vi "Get Blob Properties.vi"(8 "error in (no error)":errorcluster, 9 "Blob":string, 10 "Container":string, 11 "Azure Session in":refnum<class "Session.lvclass">) -> (0 "error out":errorcluster, 2 "Blob Properties":T1[](array[typedef]), 3 "Azure Session out":refnum<class "Session.lvclass">)   [LabVIEW 2015, in "NI_Azure_Blob.lvlib"]
doc: "Returns all system properties and user-defined metadata on the blob."
uses:
  NI_Azure_Blob.lvlib
  Core/Session/Session.lvclass
  Core/Name Value Pair.ctl
  Core/Session/Session.lvclass/Session.ctl
  Core/Session/Write HTTP Verb.vi
  Core/Session/Write URL Suffix.vi
  Core/NI_Azure_Core.lvlib
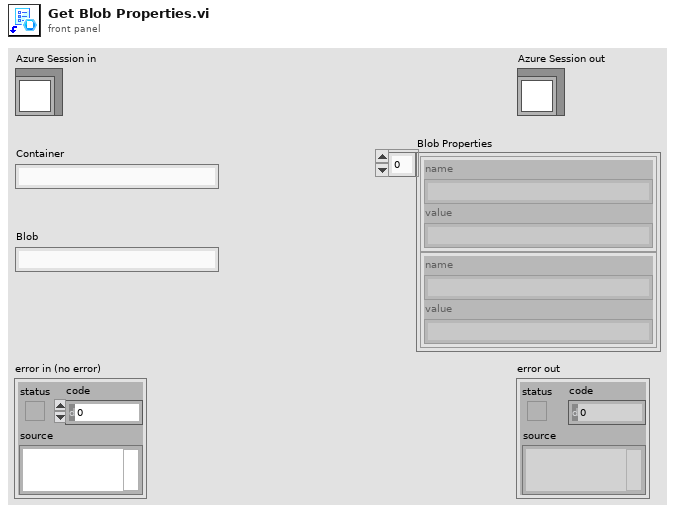
[diagram p1: front panel]
types:
  T1 = typedef "NI_Azure_Core.lvlib/Name Value Pair.ctl" = cluster{"name":string, "value":string}
  T2 = typedef "NI_Azure_Core.lvlib/Response.ctl" = cluster{"Headers":string, "Body":string}
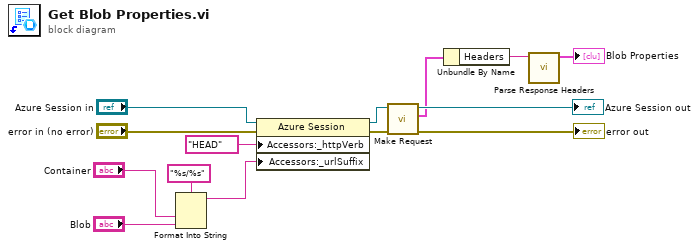
[diagram p0: block diagram]
diagram:
  n1 = Format Into String(format string="%s/%s", "Container", "Blob") -> (resulting string=w2:string)  [unwired: 2 in, 1 out]
  n2 = property class="Azure Session"(reference="Azure Session in", error in="error in (no error)", "Accessors:_httpVerb"="HEAD" ("HTTP-Verb"), "Accessors:_urlSuffix"=w2) -> (reference out=w3:refnum<class "Session.lvclass">, error out=w5:errorcluster)
  n3 = call "Make Request.vi"("error in (no error)"=w5, "Session in"=w3) -> ("error out"=→"error out":errorcluster, "Response"=w6:T2, "Session out"=→"Azure Session out":refnum<class "Session.lvclass">)  [unwired: 7 in]
  n4 = Unbundle By Name(w6) -> ("Headers"=w8:string)
  n5 = call "Parse Response Headers.vi"("String"=w8) -> ("Response Headers"=→"Blob Properties":T1[])  [unwired: 10 in]
